vi "DMAsOverflow.vi"() -> (2 "DMAsOverFlow":u16)   [LabVIEW 2013]
uses:
  GlobalReg.vi
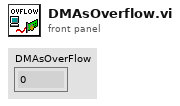
[diagram p1: front panel]
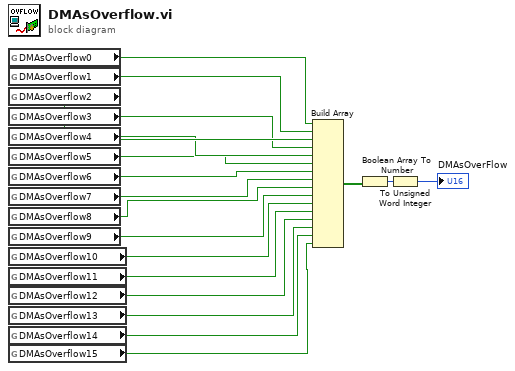
[diagram p0: block diagram]
diagram:
  n1 = global read "GlobalReg.vi" "DMAsOverflow0"() -> (w19:bool)
  n2 = global read "GlobalReg.vi" "DMAsOverflow1"() -> (w18:bool)
  n3 = global read "GlobalReg.vi" "DMAsOverflow2"() -> (w17:bool)
  n4 = global read "GlobalReg.vi" "DMAsOverflow3"() -> (w16:bool)
  n5 = global read "GlobalReg.vi" "DMAsOverflow4"() -> (w15:bool)
  n6 = global read "GlobalReg.vi" "DMAsOverflow5"() -> (w14:bool)
  n7 = global read "GlobalReg.vi" "DMAsOverflow6"() -> (w13:bool)
  n8 = global read "GlobalReg.vi" "DMAsOverflow7"() -> (w12:bool)
  n9 = global read "GlobalReg.vi" "DMAsOverflow8"() -> (w11:bool)
  n10 = global read "GlobalReg.vi" "DMAsOverflow9"() -> (w10:bool)
  n11 = global read "GlobalReg.vi" "DMAsOverflow10"() -> (w9:bool)
  n12 = global read "GlobalReg.vi" "DMAsOverflow11"() -> (w8:bool)
  n13 = global read "GlobalReg.vi" "DMAsOverflow12"() -> (w7:bool)
  n14 = global read "GlobalReg.vi" "DMAsOverflow13"() -> (w6:bool)
  n15 = global read "GlobalReg.vi" "DMAsOverflow14"() -> (w5:bool)
  n16 = global read "GlobalReg.vi" "DMAsOverflow15"() -> (w4:bool)
  n17 = Build Array(w19, w18, w17, w16, w15, w14, w13, w12, w11, w10, w9, w8, w7, w6, w5, w4) -> (w3:bool[])
  n18 = Boolean Array To Number(Boolean array=w3) -> (number=w2:u16)
  n19 = To Unsigned Word Integer(number=w2) -> (unsigned 16bit integer=→"DMAsOverFlow":u16)
